vi "APTpiezoSet.vi"(7 "Set position":sgl min=0 max=500, 8 "error in (no error)":errorcluster, 11 "reference":refnum<k7>) -> (0 "error out":errorcluster, 3 "reference out":refnum<k7>)   [LabVIEW 2015]
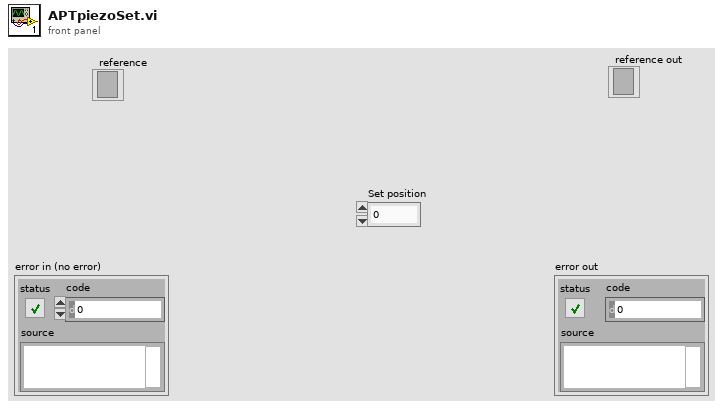
[diagram p1: front panel]
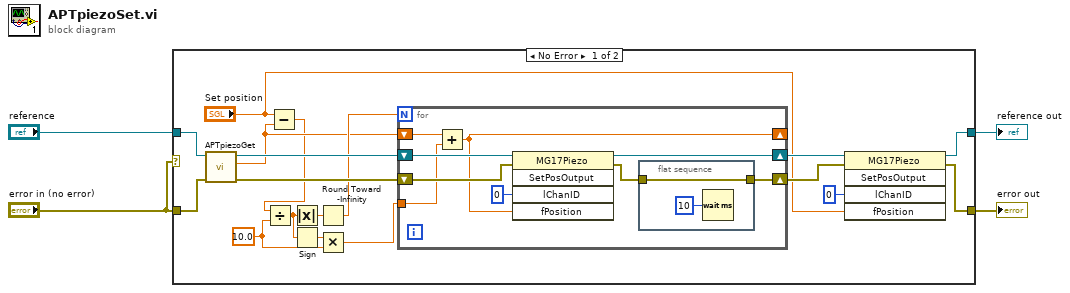
[diagram p0: block diagram]
diagram:
  n1 = case shown="No Error" "error in (no error)" {
    tunnel: [w14 w35] -> w4
    tunnel: [w16 w34] -> w3
    tunnel: "reference" -> [w22 w35]
    tunnel: "error in (no error)" -> [w19 w34]
    frame No Error {
      w8 = sgl 10.0 ("y")
      n2 = call "APTpiezoGet.vi"("error in (no error)"=w19, "reference"=w22) -> ("error out"=w20:errorcluster, "pfPosition"=w7:sgl, "reference out"=w21:refnum<k7>)  [unwired: 7 in]
      n3 = Subtract(x="Set position", y=w7) -> (x-y=w5:sgl)
      n4 = Divide(x=w5, y=w8) -> (x/y=w11:sgl)
      n5 = Absolute Value(x=w11) -> (abs(x)=w12:sgl)
      n6 = Sign(1:w11) -> (0:w10:sgl)
      n7 = Round Toward -Infinity(1:w12) -> (0:w18:sgl)
      n8 = Multiply(x=w10, y=w8) -> (x*y=w9:sgl)
      n9 = for {
        N: w18 -> [_]
        shift-right: [w31] -> w15
        shift-left: w21 -> [w29]
        shift-right: [w26] -> w17
        shift-left: w20 -> [w28]
        shift-right: [w23] -> _
        shift-left: w7 -> [w25]
        tunnel: w9 -> [w24]
        n10 = Add(x=w25, y=w24) -> (x+y=w23:sgl)
        n11 = invoke class="MG17Piezo" method="SetPosOutput"(reference=w29, error in=w28, "lChanID"=0, "fPosition"=w23) -> (reference out=w31:refnum<k7>, error out=w27:errorcluster)  [unwired: 1 in, 3 out]
        n12 = flat-sequence {
          tunnel: [w32] -> w26
          tunnel: w27 -> [w32]
          frame #0 {
            n13 = Wait (ms)(milliseconds to wait=u32 10) -> ()  [unwired: 1 out]
          }
        }
      }
      n14 = invoke class="MG17Piezo" method="SetPosOutput"(reference=w15, error in=w17, "lChanID"=0, "fPosition"="Set position") -> (reference out=w14:refnum<k7>, error out=w16:errorcluster)  [unwired: 1 in, 3 out]
    }
    frame Error {
    }
  }
  "error out" <- w3
  "reference out" <- w4
